vi "Untitled 2.vi"(0 "error in (no error)":errorcluster) -> (8 "error out":errorcluster)   [LabVIEW 2014]
panel:
  in  "Boolean":bool
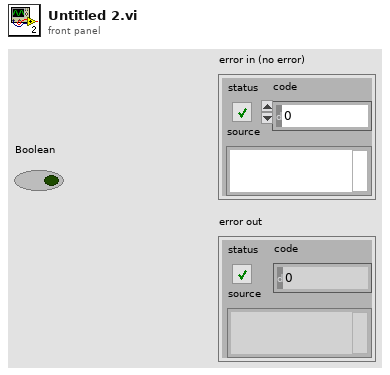
[diagram p1: front panel]
types:
  T1 = typedef "WPI_MotorControlDeviceRef.ctl" = cluster{"DeviceStatus":errorcluster, "Type":T2, "PWM":cluster{"Controller":T3, "PWM Channel":T4, "DeadBand":T5}, "CAN":cluster{"Device Number":u8, "Control Mode":T6, "Semaphore":T7, "Max Vout":dbl, "TalonSRX Control Mode":T8}, "Invert":bool, "TransformRef":T9, "InvTransformRef":T9}
  T2 = typedef "WPI_MotorControlType.ctl" = enum16{"PWM", "CAN", "CANTalonSRX"}
  T3 = typedef "FPGA_TypedefDigitalModule.ctl" = enum16{"Controller 1"}
  T4 = typedef "FPGA_DIOPWMChannel.ctl" = enum8{"PWM 0", "PWM 1", "PWM 2", "PWM 3", "PWM 4", "PWM 5", "PWM 6", "PWM 7", "PWM 8", "PWM 9", "PWM MXP 0", "PWM MXP 1", "PWM MXP 2", "PWM MXP 3", "PWM MXP 4", "PWM MXP 5", "PWM MXP 6", "PWM MXP 7", "PWM MXP 8", "PWM MXP 9", "Invalid"}
  T5 = typedef "WPI_PWMDeadband.ctl" = cluster{"Name":string, "maxPositivePwm":i32, "minPositivePwm":i32, "centerPwm":i32, "maxNegativePwm":i32, "minNegativePwm":i32, "angularRange":u16}
  T6 = typedef "WPI_CANJaguar_ControlMode.ctl" = enum8{"Percent VBus", "Current", "Speed", "Position", "Voltage"}
  T7 = typedef "Semaphore RefNum" = refnum<k1>
  T8 = typedef "WPI_CANTalonSRX_APIControlMode.ctl" = enum8{"Percent VBus", "Speed", "Position", "Slave", "Unchanged / Invalid"}
  T9 = typedef "WPI_PWMTransform_ConPane.ctl" = refnum<vi>
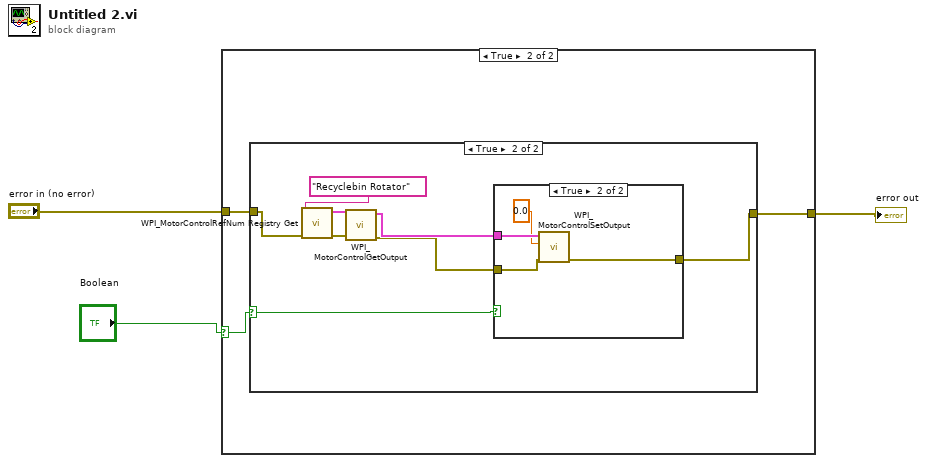
[diagram p0: block diagram]
diagram:
  n1 = case shown="True" "Boolean" {
    selector: "Boolean" -> [_ w5]
    tunnel: "error in (no error)" -> [w4 w6]
    tunnel: [w4 w7] -> w2
    frame False {
    }
    frame True {
      n2 = case shown="True" w5 {
        selector: w5 -> [_ w9]
        tunnel: [w8 w10] -> w7
        tunnel: w6 -> [w8 w13]
        frame False {
        }
        frame True {
          n3 = call <vilib>:"WPI_MotorControlRefNum Registry Get.vi"("error in (no error)"=w13, "refnum name"="Recyclebin Rotator") -> ("error out"=w16:errorcluster, "MotorControlDevRef"=w14:T1)  [unwired: 8 in]
          n4 = call <vilib>:"WPI_MotorControlGetOutput.vi"("error in (no error)"=w16, "MotorControlDevRef"=w14) -> ("error out"=w11:errorcluster, "MotorControlDevRef"=w12:T1)  [unwired: 7 in, 1 out]
          n5 = case shown="True" w9 {
            tunnel: [w17 w21] -> w10
            tunnel: w12 -> [_ w20]
            tunnel: w11 -> [w17 w18]
            frame False {
            }
            frame True {
              n6 = call <vilib>:"WPI_MotorControlSetOutput.vi"("error in (no error)"=w18, "Output"=0.0, "MotorControlDevRef"=w20) -> ("error out"=w21:errorcluster)  [unwired: 6 in, 2 out]
            }
          }
        }
      }
    }
  }
  "error out" <- w2
